vi "Get all tests.vi"(8 "error in (no error)":errorcluster, 11 "Test Case in":refnum<class "LUnit Test Case.lvclass">) -> (0 "error out":errorcluster, 2 "VI refs out":refnum<vi>[](array[refnum]), 3 "Test Case out":refnum<class "LUnit Test Case.lvclass">)   [LabVIEW 2020, in "Slave Test Runner.lvclass"]
uses:
  Slave Test Runner.lvclass
  Test Case/LUnit Test Case.lvclass
  Test Case/LUnit Test Case.lvclass/LUnit Test Case.ctl
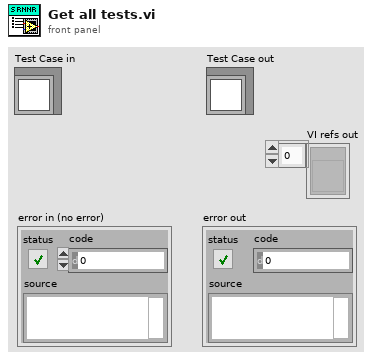
[diagram p1: front panel]
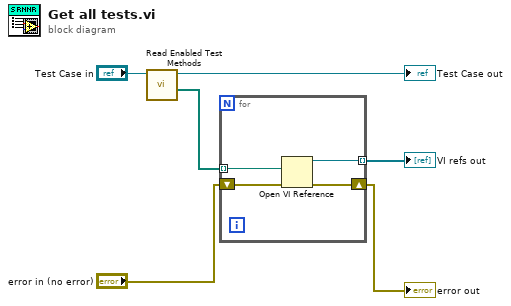
[diagram p0: block diagram]
diagram:
  n1 = call "Read Enabled Test Methods.vi"("LUnit Test Case In"="Test Case in") -> ("Paths"=w4:path[], "LUnit Test Case Out"=→"Test Case out":refnum<class "LUnit Test Case.lvclass">)  [unwired: 8 in, 1 out]
  n2 = for {
    tunnel: w4 -> [w10] mode=indexing
    shift-right: [w8] -> w3
    shift-left: "error in (no error)" -> [w9]
    tunnel: [w7] -> w2 mode=indexing
    n3 = Open VI Reference(vi path=w10, error in (no error)=w9) -> (vi reference=w7:refnum<vi>, error out=w8:errorcluster)  [unwired: 4 in]
  }
  "error out" <- w3
  "VI refs out" <- w2
